vi "Lockin.DAQ.EventRegistration.vi"(8 "error in (no error)":errorcluster, 10 "DAQmx in":refnum<event-registration>, 11 "Lockin.DAQ in":refnum<class "Lockin.DAQ.lvclass">) -> (0 "error out":errorcluster, 2 "DAQmx out":refnum<event-registration>, 3 "Lockin.DAQ out":refnum<class "Lockin.DAQ.lvclass">)   [LabVIEW 2016, in "Lockin.DAQ.lvclass"]
uses:
  Lockin.DAQ.lvclass
  Lockin.DAQ.lvclass/Lockin.DAQ.ctl
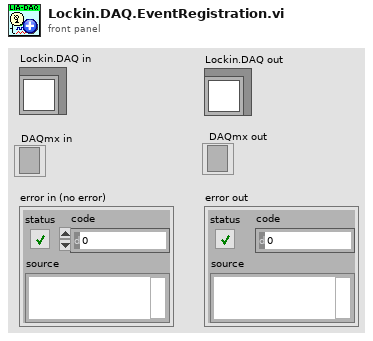
[diagram p1: front panel]
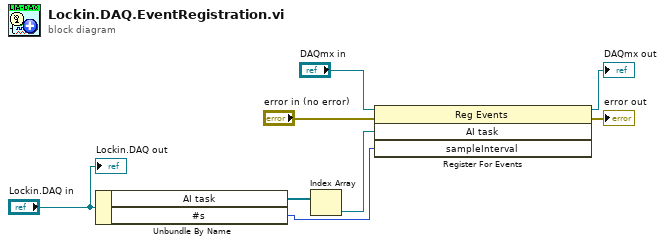
[diagram p0: block diagram]
diagram:
  n1 = Unbundle By Name("Lockin.DAQ in") -> ("AI task"=w6:refnum<k21>[], "#s"=w5:i32)
  n2 = Index Array(array=w6) -> (element=w3:refnum<k21>)  [unwired: 1 in]
  n3 = register-events(reference="DAQmx in", error in="error in (no error)", w3, w5) -> (reference out=→"DAQmx out":refnum<event-registration>, error out=→"error out":errorcluster)
  "Lockin.DAQ out" <- "Lockin.DAQ in"
